vi "Read Igus CanOpen.vi"(6 "Sub Index":u8 format="%.0x", 8 "error in (no error)":errorcluster, 10 "Address":u16 format="%.0x", 11 "MB session in":refnum<class "MB_Master.lvclass">) -> (0 "error out":errorcluster, 1 "Command":T1={"Function Code"=1, "Data"=[], "RTU_DataBytes"=0} {"Data" format="%.0x"}, 2 "Response":T1={"Function Code"=1, "Data"=[], "RTU_DataBytes"=0} {"Data" format="%.0x"}, 3 "MB session out":refnum<class "MB_Master.lvclass">)   [LabVIEW 2016, in "MB Master.lvlib"]
doc: "Function Code 43 / 14: Read device ID objects. Specify the type of access using the <b>read device ID code</b> and the id of the starting object using <b>object ID</b>.\n\nread device ID codes:\n 0x01 - Basic: Request the basic stream of devID objects (0x00 to 0x02) starting from the specified object ID.\n 0x02 - Regular: Requests the regular stream of devID objects (0x00 to 0x7F) starting from the specified object ID.\n 0x03 - Extended: Requests the extended stream of devID objects (0x00 to 0xFF) starting from the specified object ID.\n 0x04 - Single: Requests a single devID object specified by object ID.\n\nResponse is an array of devID objects. Each element contains the object ID and string value. The conformity level indicates the type of access supported by the device.\n\nConformity level values:\n0x01 - Basic (stream only)\n0x02 - Regular (stream only)\n0x03 - Extended (stream only)\n0x81 - Basic (stream and single)\n0x82 - Regular (stream and single)\n0x83 - Extended (stream and single)"
uses:
  MB Master.lvlib
  MB_Master.lvclass
  MB_PDU/MB_PDU_Cluster.ctl
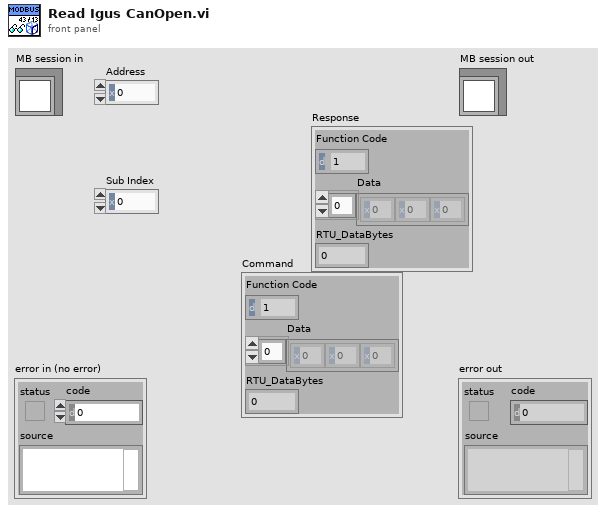
[diagram p1: front panel]
types:
  T1 = typedef "MB Master.lvlib/MB_PDU_Cluster.ctl" = cluster{"Function Code":u8, "Data":u8[], "RTU_DataBytes":i32}
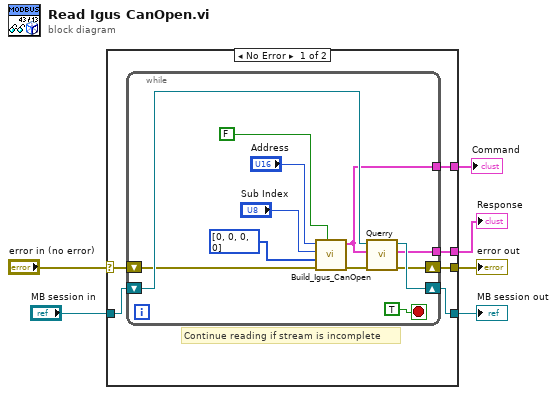
[diagram p0: block diagram]
diagram:
  n1 = case shown="No Error" "error in (no error)" {
    selector: "error in (no error)" -> [w10 w26]
    tunnel: [w9 w26] -> w5
    tunnel: [w12 w25] -> w3
    tunnel: "MB session in" -> [w11 w25]
    tunnel: [w8 _] -> w2
    tunnel: [w7 _] -> w1
    frame No Error {
      # "Continue reading if stream is incomplete"
      n2 = while {
        shift-right: [w19] -> w9
        shift-left: w10 -> [w20]
        shift-right: [w24] -> w12
        shift-left: w11 -> [w23]
        tunnel: [w18] -> w8
        tunnel: [w13] -> w7
        stop <- TRUE stop-if-true
        n3 = call "Build_Igus_CanOpen.vi"("Read (F) / Write"=FALSE, "error in (no error)"=w20, "Data [1-4]"=u8[] [0, 0, 0, 0], "Sub Index"="Sub Index", "Address"="Address") -> ("error out"=w21:errorcluster, "MB_PDU"=w13:T1)  [unwired: 5 in]
        n4 = call-dynamic "Querry.vi"("error in (no error)"=w21, "PDU_req"=w13, "MB_Master in"=w23) -> ("error out"=w19:errorcluster, "PDU_resp"=w18:T1, "MB_Master out"=w24:refnum<class "MB_Master.lvclass">)  [unwired: 6 in]
      }
    }
    frame Error {
    }
  }
  "error out" <- w5
  "MB session out" <- w3
  "Response" <- w2
  "Command" <- w1
